vi "HelloWorld.vi"() -> ()   [LabVIEW 2019]
panel:
  out "Output string":string
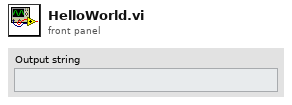
[diagram p1: front panel]
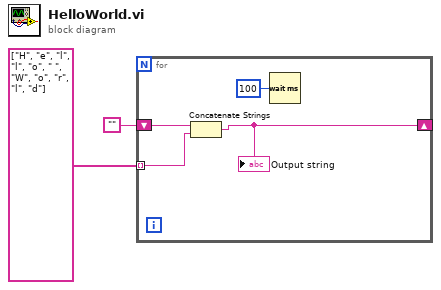
[diagram p0: block diagram]
diagram:
  n1 = for {
    tunnel: string[] ["H", "e", "l", "l", "o", " ", "W", "o", "r", "l", "d"] ("Array") -> [w5] mode=indexing
    shift-right: [w4] -> _
    shift-left: "" -> [w6]
    n2 = Concatenate Strings(w6, w5) -> (w4:string)
    "Output string" <- w4
    n3 = Wait (ms)(milliseconds to wait=u32 100) -> ()  [unwired: 1 out]
  }
